vi "A4_Taladro.vi"() -> ()   [LabVIEW 2025]
panel:
  out "Taladro":u8(slide) scale=0.0..100.0
  out "Piezas delgadas":dbl
  out "Piezas gruesas":dbl
  in  "Arranque":bool
  in  "Sensor SH":bool
  out "Posición A3":bool
  out "Posición A0":bool
  out "Posición  A1":bool
  out "Posición A2":bool
  in  "PARO":bool
  # "Apagado"
  # "Encendido"
  # "Verde para pieza gruesa.\n\nAzul para pieza delgada."
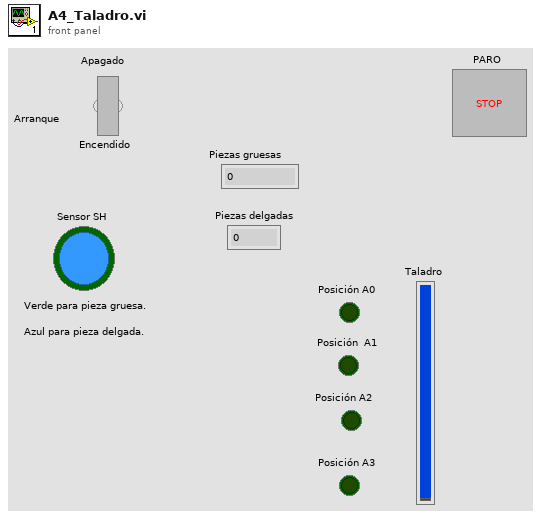
[diagram p1: front panel]
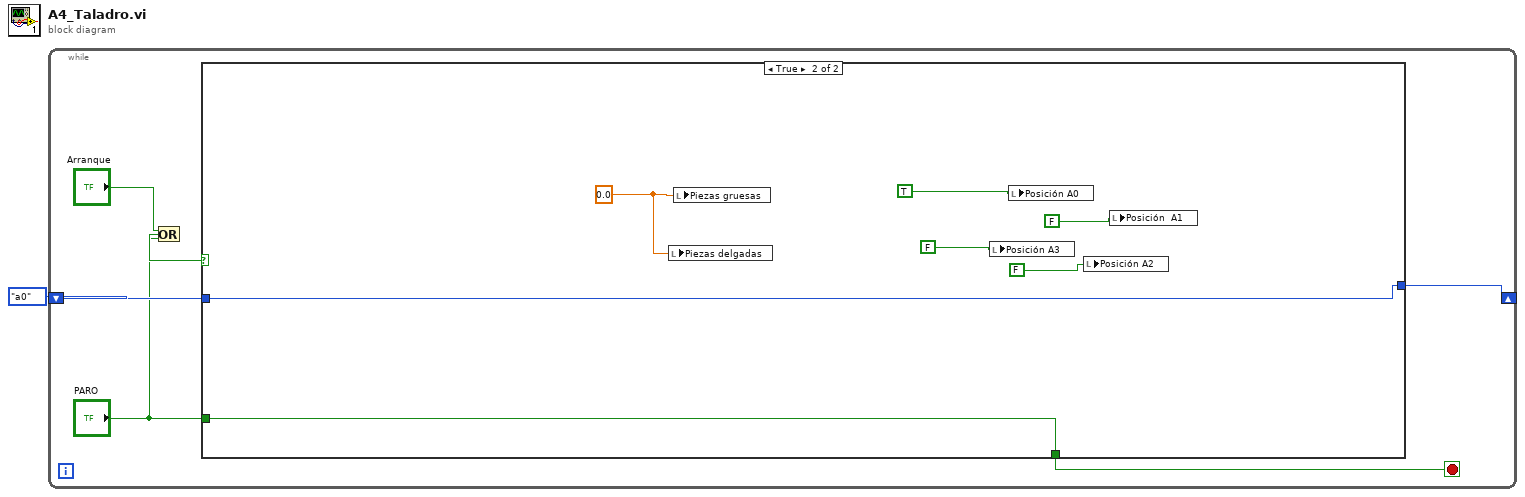
[diagram p0: block diagram]
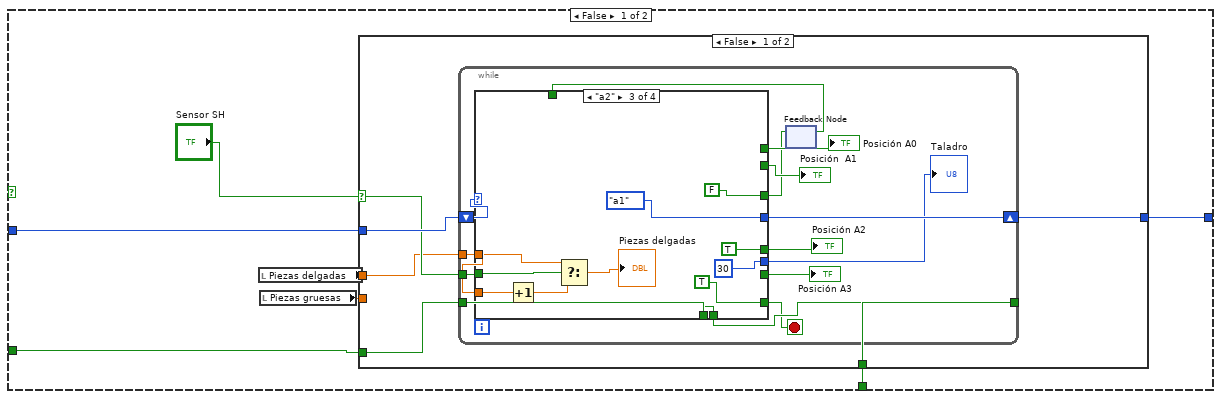
[diagram p2: hidden frame]
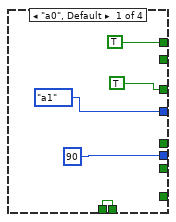
[diagram p3: hidden frame]
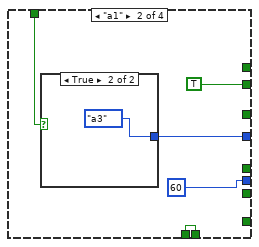
[diagram p4: hidden frame]
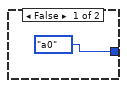
[diagram p5: hidden frame]
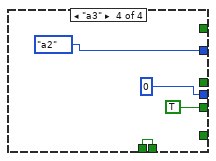
[diagram p6: hidden frame]
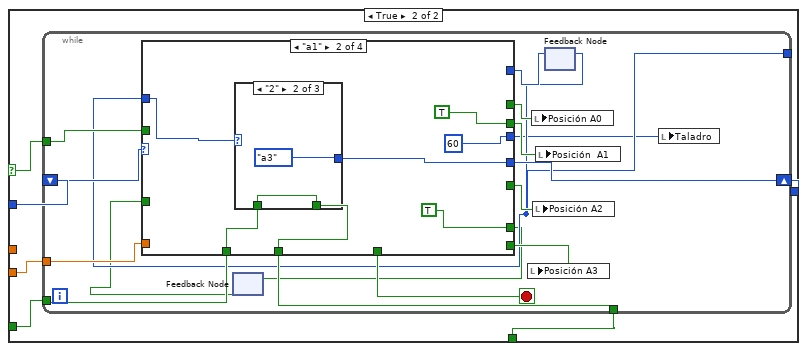
[diagram p7: hidden frame]
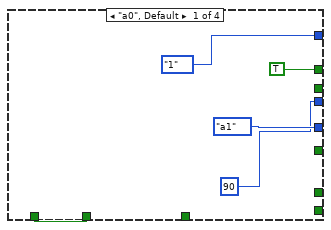
[diagram p8: hidden frame]
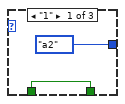
[diagram p9: hidden frame]
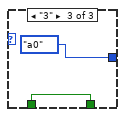
[diagram p10: hidden frame]
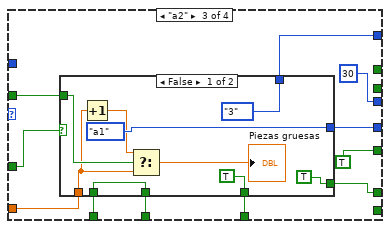
[diagram p11: hidden frame]
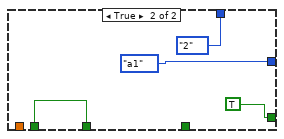
[diagram p12: hidden frame]
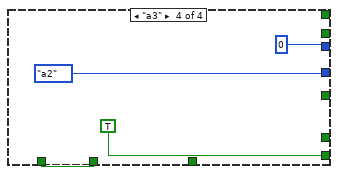
[diagram p13: hidden frame]
diagram:
  n1 = while {
    shift-right: [w6] -> _
    shift-left: enum16{"a0", "a1", "a2", "a3"}."a0" -> [w7]
    stop <- w5 stop-if-true
    n2 = Or(x="Arranque", y="PARO") -> (x .or. y?=w4:bool)
    n3 = case shown="True" w4 {
      tunnel: w7 -> [w14 w135]
      tunnel: [w11 w135] -> w6
      tunnel: [w13 w136] -> w5
      tunnel: "PARO" -> [w12 w136]
      frame False {
        n4 = local read "Piezas delgadas"() -> (w9:dbl)
        n5 = local read "Piezas gruesas"() -> (w10:dbl)
        n6 = case shown="False" "Sensor SH" {
          selector: "Sensor SH" -> [w16 w63]
          tunnel: [w19 w66] -> w11
          tunnel: w14 -> [w20 w67]
          tunnel: [w18 w64] -> w13
          tunnel: w12 -> [w17 w65]
          tunnel: w10 -> [_ w62]
          tunnel: w9 -> [w15 _]
          frame False {
            n7 = while {
              tunnel: w15 -> [w29]
              shift-right: [w33] -> w19
              shift-left: w20 -> [w34]
              tunnel: w17 -> [w31]
              tunnel: [w32] -> w18
              tunnel: w16 -> [w30]
              stop <- w28 stop-if-true
              n8 = feedback #1() -> (w22:bool)  [unwired: 1 in]
              n9 = case shown="\"a2\"" w34 {
                tunnel: [enum16{"a0", "a1", "a2", "a3"}."a1" w43 enum16{"a0", "a1", "a2", "a3"}."a1" enum16{"a0", "a1", "a2", "a3"}."a2"] -> w33
                tunnel: [TRUE ("Posición A0") _ _ _] -> w27
                tunnel: [_ TRUE ("Posición  A1") _ _] -> w26
                tunnel: [_ _ TRUE ("Posición A2") _] -> w25
                tunnel: [_ _ _ TRUE ("Posición A3")] -> w24
                tunnel: [w37 w42 w55 w59] -> w32
                tunnel: w31 -> [w37 w42 w55 w59]
                tunnel: w30 -> [_ _ w53 _]
                tunnel: w29 -> [_ _ w52 _]
                tunnel: w29 -> [_ _ w50 _]
                tunnel: [_ _ TRUE _] -> w28
                tunnel: [TRUE _ FALSE _] -> w23
                tunnel: w22 -> [_ w41 _ _]
                tunnel: [90 60 30 0] -> w21
                frame "a0", Default {
                }
                frame "a1" {
                  n10 = case shown="True" w41 {
                    tunnel: [enum16{"a0", "a1", "a2", "a3"}."a0" enum16{"a0", "a1", "a2", "a3"}."a3"] -> w43
                    frame False {
                    }
                    frame True {
                    }
                  }
                }
                frame "a2" {
                  n11 = Increment(x=w50) -> (x+1=w51:dbl)
                  n12 = Select(t=w52, s=w53, f=w51) -> (s? t:f=→"Piezas delgadas":dbl)
                }
                frame "a3" {
                }
              }
              "Posición A0" <- w27
              "Posición  A1" <- w26
              "Posición A2" <- w25
              "Posición A3" <- w24
              "Taladro" <- w21
              n13 = feedback-in #1(w23) -> ()
            }
          }
          frame True {
            n14 = while {
              tunnel: [w71] -> _
              tunnel: w62 -> [w78]
              shift-right: [w82] -> w66
              shift-left: w67 -> [w83]
              tunnel: w63 -> [w79]
              tunnel: w65 -> [w81]
              tunnel: [w80] -> w64
              stop <- w77 stop-if-true
              n15 = feedback #2() -> (w69:bool)  [unwired: 1 in]
              n16 = feedback #3() -> (w71:enum16{"1", "2", "3"})  [unwired: 1 in]
              n17 = case shown="\"a1\"" w83 {
                tunnel: [TRUE ("Posición A0") _ _ _] -> w76
                tunnel: [enum16{"a0", "a1", "a2", "a3"}."a1" w93 w112 enum16{"a0", "a1", "a2", "a3"}."a2"] -> w82
                tunnel: [_ TRUE ("Posición  A1") _ _] -> w75
                tunnel: w71 -> [_ w94 _ _]
                tunnel: [enum16{"1", "2", "3"}."1" _ w104 _] -> w72
                tunnel: w69 -> [_ _ w111 _]
                tunnel: [_ TRUE w103 _] -> w70
                tunnel: [_ _ _ TRUE ("Posición A3")] -> w73
                tunnel: [_ _ TRUE ("Posición A2") _] -> w74
                tunnel: w81 -> [w86 w92 w109 w127]
                tunnel: [w86 w91 w108 w127] -> w80
                tunnel: w79 -> [_ _ w107 _]
                tunnel: w78 -> [_ _ w106 _]
                tunnel: [_ _ w105 _] -> w77
                tunnel: [u8 90 ("Taladro") u8 60 ("Taladro") u8 30 ("Taladro") u8 0 ("Taladro")] -> w68
                frame "a0", Default {
                }
                frame "a1" {
                  n18 = case shown="\"2\"" w94 {
                    tunnel: [enum16{"a0", "a1", "a2", "a3"}."a2" enum16{"a0", "a1", "a2", "a3"}."a3" enum16{"a0", "a1", "a2", "a3"}."a0"] -> w93
                    tunnel: [w96 w99 w101] -> w91
                    tunnel: w92 -> [w96 w99 w101]
                    frame "1" {
                    }
                    frame "2" {
                    }
                    frame "3" {
                    }
                  }
                }
                frame "a2" {
                  n19 = case shown="False" w111 {
                    tunnel: [enum16{"a0", "a1", "a2", "a3"}."a1" enum16{"a0", "a1", "a2", "a3"}."a1"] -> w112
                    tunnel: [w117 w124] -> w108
                    tunnel: w109 -> [w117 w124]
                    tunnel: w107 -> [w120 _]
                    tunnel: w106 -> [w118 _]
                    tunnel: [TRUE _] -> w105
                    tunnel: [enum16{"1", "2", "3"}."3" enum16{"1", "2", "3"}."2"] -> w104
                    tunnel: [TRUE TRUE] -> w103
                    frame False {
                      n20 = Increment(x=w118) -> (x+1=w119:dbl)
                      n21 = Select(t=w119, s=w120, f=w118) -> (s? t:f=→"Piezas gruesas":dbl)
                    }
                    frame True {
                    }
                  }
                }
                frame "a3" {
                }
              }
              n22 = feedback-in #2(w70) -> ()
              n23 = local write "Posición A3"(w73) -> ()
              n24 = local write "Posición A0"(w76) -> ()
              n25 = local write "Posición A2"(w74) -> ()
              n26 = local write "Posición  A1"(w75) -> ()
              n27 = feedback-in #3(w72) -> ()
              n28 = local write "Taladro"(w68) -> ()
            }
          }
        }
      }
      frame True {
        w134 = 0.0 ("Piezas gruesas")
        n29 = local write "Piezas delgadas"(w134) -> ()
        n30 = local write "Piezas gruesas"(w134) -> ()
        n31 = local write "Posición A3"(FALSE ("Posición A3")) -> ()
        n32 = local write "Posición A0"(TRUE ("Posición A0")) -> ()
        n33 = local write "Posición A2"(FALSE ("Posición A2")) -> ()
        n34 = local write "Posición  A1"(FALSE ("Posición  A1")) -> ()
      }
    }
  }
